vi "CheckParameters.vi"(8 "error in (no error)":errorcluster, 10 "Parameters":u32[](array[numeric]), 11 "Burst in":refnum<class "Burst.lvclass">) -> (0 "error out":errorcluster, 3 "Burst out":refnum<class "Burst.lvclass">)   [LabVIEW 2013, in "Burst.lvclass"]
uses:
  Burst.lvclass
  TestInterface/TestInterface.lvclass
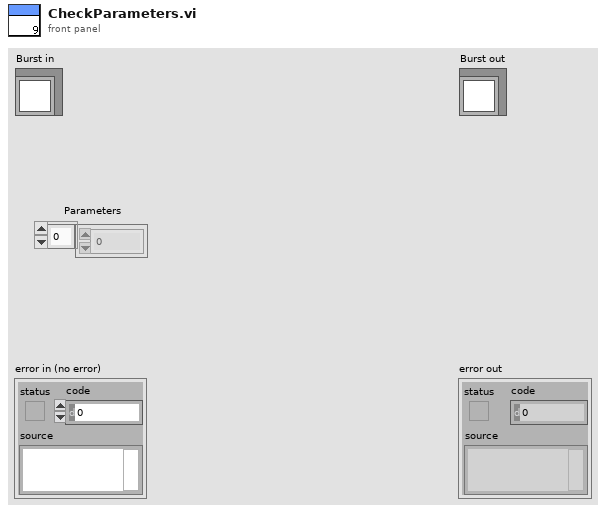
[diagram p1: front panel]
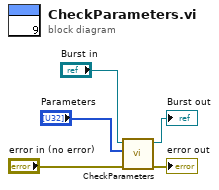
[diagram p0: block diagram]
diagram:
  n1 = call-parent "CheckParameters.vi"("error in (no error)"="error in (no error)", "Parameters"="Parameters", "TestInterface in"="Burst in") -> ("error out"=→"error out":errorcluster, "TestInterface out"=→"Burst out":refnum<class "Burst.lvclass">)  [unwired: 7 in]
